vi "exv valves.vi"(0 "Large Gas Cluster":T8, 1 "Medium Gas Cluster":T7, 3 "Small Gas Cluster":T6, 4 "Large Liquid Cluster":T5, 5 "Medium Liquid Cluster":T4, 7 "Small Liquid Cluster":T3, 8 "Tonnage":dbl, 9 "Desired Psuc":dbl, 10 "Reinitialize Controller P":bool, 11 "Controller Toggle P":bool, 12 "Tonnage Threshold":dbl=40.0 format="%#_13g", 13 "Desired Tsuc":dbl, 14 "Delta P Threshold":dbl=5.0 format="%#_13g", 15 "Current Psuc":dbl format="%#_13g", 16 "Delta T Threshold":dbl=5.0 format="%#_13g", 17 "Current Tsuc":dbl format="%#_13g", 18 "Reinitialize Controller T":bool, 19 "Controller Toggle T":bool) -> (20 "Gas Valves Output":T2, 27 "Liquid Valves Output":T1)   [LabVIEW 2017]
doc: "Control logic for all controllers on liquid and gas lines. Thresholding procedure that determines which controller should be operating based on current process variable. Passes the chosen controller to the PID vi's"
panel:
  out "output to valve 3":dbl
  out "output to valve 2":dbl
  out "output to valve":dbl
  out "PID gains out small Liquid":T9
  out "Small Liquid Tuning Complete":bool
  out "Small Liquid Output":dbl(slide) scale=0.0..100.0 scale format="%#_3g"
  out "PID gains out Medium Liquid":T9
  out "Medium Liquid Tuning Complete":bool
  out "Medium Liquid Output":dbl(slide) scale=0.0..100.0 scale format="%#_3g"
  out "PID gains out large liquid":T9
  out "Large Liquid Tuning Complete":bool
  out "Large Liquid Output":dbl(slide) scale=0.0..100.0 scale format="%#_3g"
  out "PID gains out small gas":T9
  out "Small Gas Tuning Complete":bool
  out "Small Gas Output":dbl(slide) scale=0.0..100.0 scale format="%#_3g"
  out "PID gains out Medium gas":T9
  out "Medium Gas Tuning Complete":bool
  out "Medium Gas Output":dbl(slide) scale=0.0..100.0 scale format="%#_3g"
  out "PID gains out large gas":T9
  out "Large Gas Tuning Complete":bool
  out "Large Gas Output":dbl(slide) scale=0.0..100.0 scale format="%#_3g"
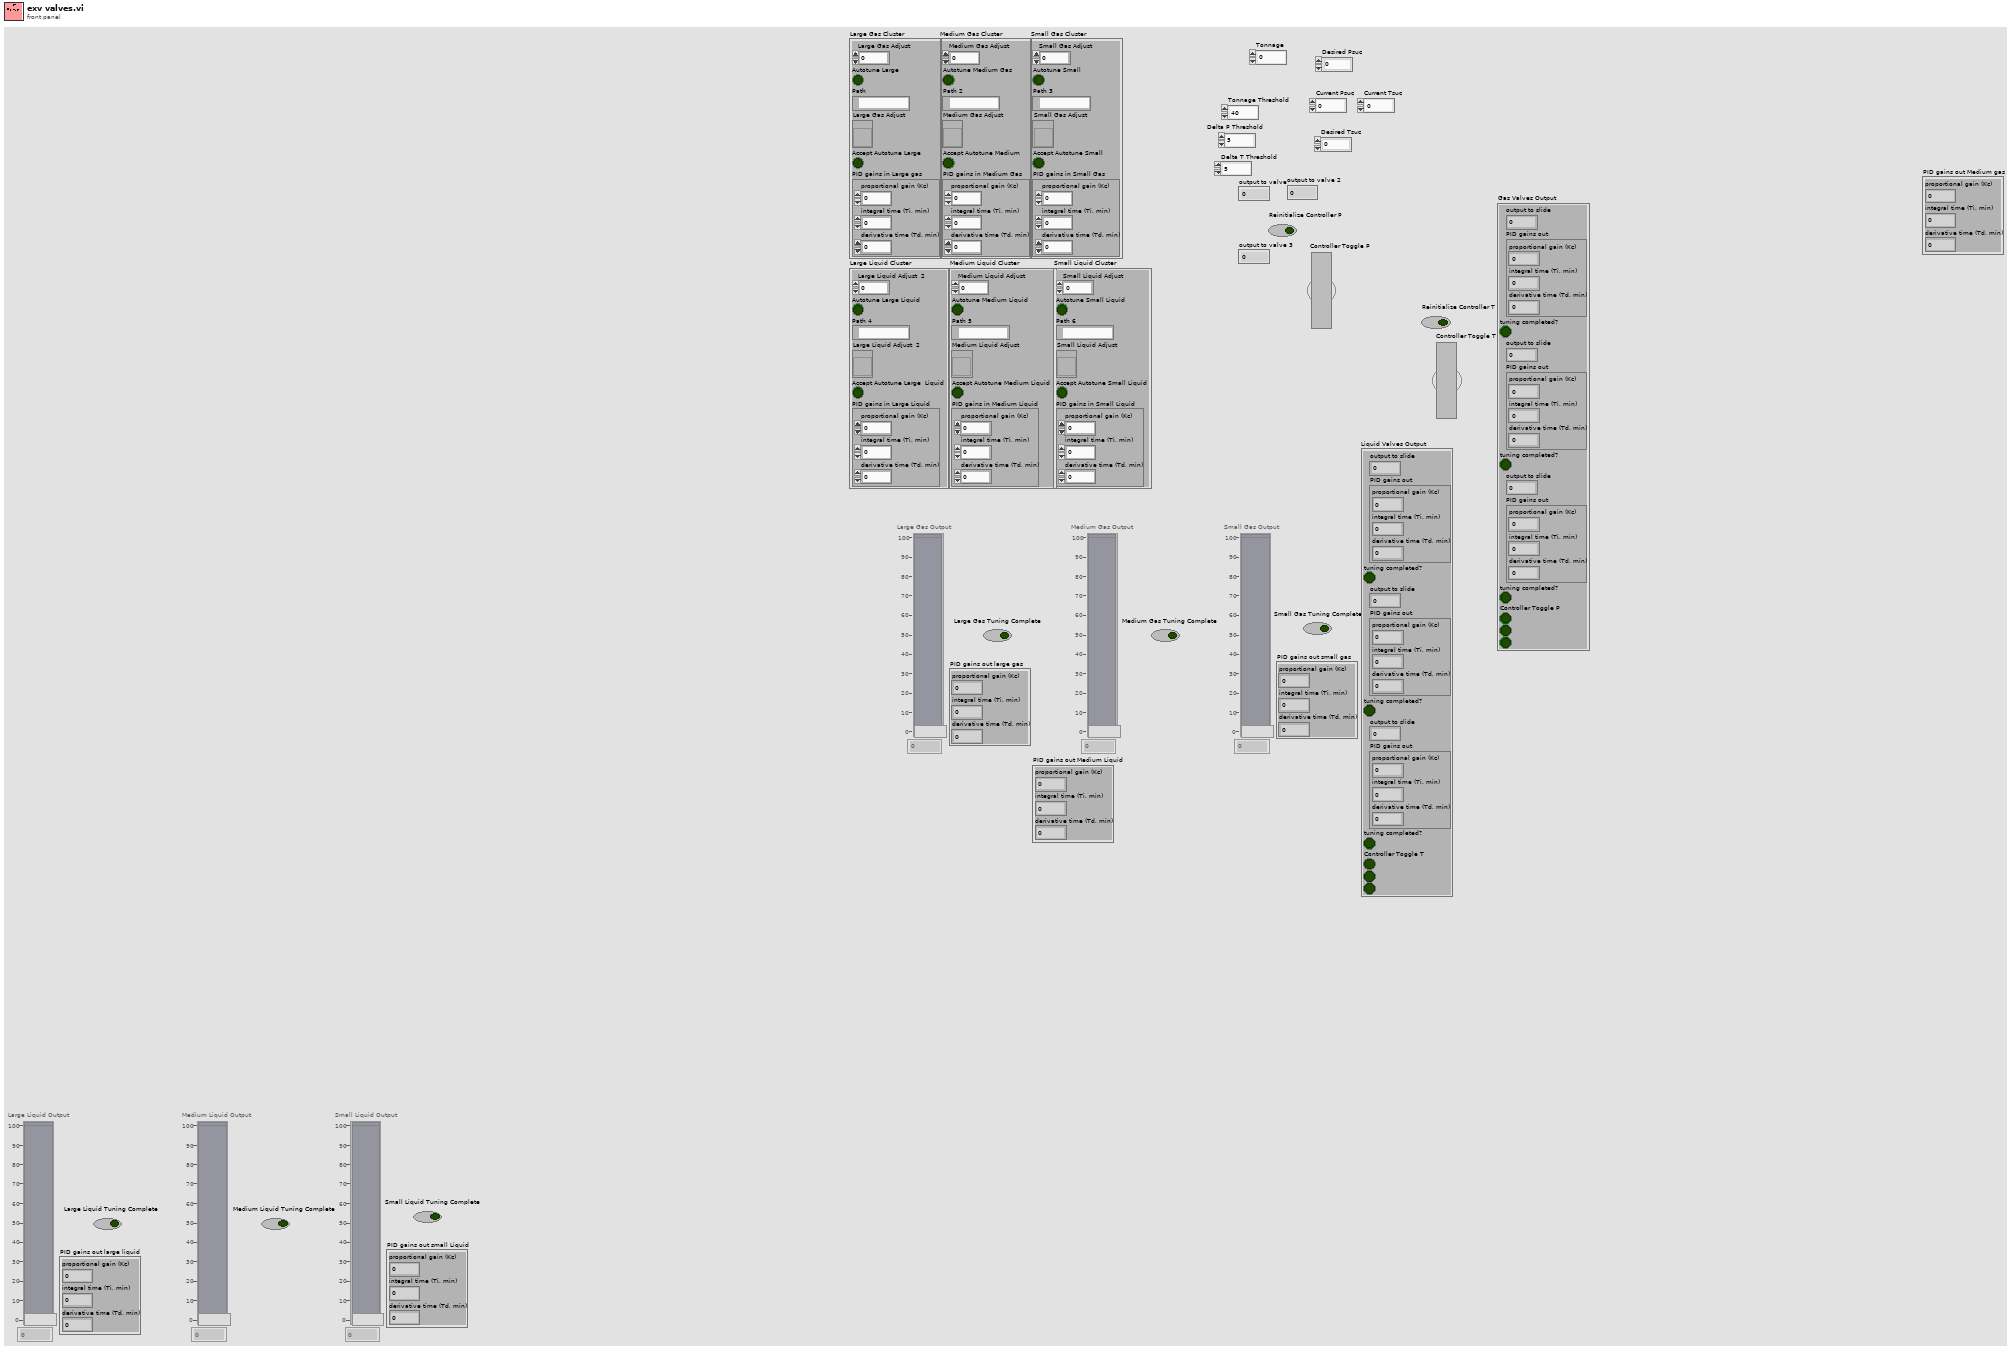
[diagram p1: front panel]
types:
  T1 = cluster{"output to slide":dbl, "PID gains out":cluster{"proportional gain (Kc)":dbl, "integral time (Ti, min)":dbl, "derivative time (Td, min)":dbl}, "tuning completed?":bool, "output to slide":dbl, "PID gains out":cluster{"proportional gain (Kc)":dbl, "integral time (Ti, min)":dbl, "derivative time (Td, min)":dbl}, "tuning completed?":bool, "output to slide":dbl, "PID gains out":cluster{"proportional gain (Kc)":dbl, "integral time (Ti, min)":dbl, "derivative time (Td, min)":dbl}, "tuning completed?":bool, "Controller Toggle T":bool, bool, bool}
  T2 = cluster{"output to slide":dbl, "PID gains out":cluster{"proportional gain (Kc)":dbl, "integral time (Ti, min)":dbl, "derivative time (Td, min)":dbl}, "tuning completed?":bool, "output to slide":dbl, "PID gains out":cluster{"proportional gain (Kc)":dbl, "integral time (Ti, min)":dbl, "derivative time (Td, min)":dbl}, "tuning completed?":bool, "output to slide":dbl, "PID gains out":cluster{"proportional gain (Kc)":dbl, "integral time (Ti, min)":dbl, "derivative time (Td, min)":dbl}, "tuning completed?":bool, "Controller Toggle P":bool, bool, bool}
  T3 = cluster{"Small Liquid Adjust ":dbl, "Autotune Small Liquid":bool, "Path 6":path, "Small Liquid Adjust ":refnum<vi>, "Accept Autotune Small Liquid":bool, "PID gains in Small Liquid":cluster{"proportional gain (Kc)":dbl, "integral time (Ti, min)":dbl, "derivative time (Td, min)":dbl}}
  T4 = cluster{"Medium Liquid Adjust":dbl, "Autotune Medium Liquid":bool, "Path 5":path, "Medium Liquid Adjust":refnum<vi>, "Accept Autotune Medium Liquid":bool, "PID gains in Medium Liquid":cluster{"proportional gain (Kc)":dbl, "integral time (Ti, min)":dbl, "derivative time (Td, min)":dbl}}
  T5 = cluster{"Large Liquid Adjust  2":dbl, "Autotune Large Liquid":bool, "Path 4":path, "Large Liquid Adjust  2":refnum<vi>, "Accept Autotune Large  Liquid":bool, "PID gains in Large Liquid":cluster{"proportional gain (Kc)":dbl, "integral time (Ti, min)":dbl, "derivative time (Td, min)":dbl}}
  T6 = cluster{"Small Gas Adjust":dbl, "Autotune Small":bool, "Path 3":path, "Small Gas Adjust":refnum<vi>, "Accept Autotune Small":bool, "PID gains in Small Gas ":cluster{"proportional gain (Kc)":dbl, "integral time (Ti, min)":dbl, "derivative time (Td, min)":dbl}}
  T7 = cluster{"Medium Gas Adjust":dbl, "Autotune Medium Gas":bool, "Path 2":path, "Medium Gas Adjust":refnum<vi>, "Accept Autotune Medium":bool, "PID gains in Medium Gas":cluster{"proportional gain (Kc)":dbl, "integral time (Ti, min)":dbl, "derivative time (Td, min)":dbl}}
  T8 = cluster{"Large Gas Adjust ":dbl, "Autotune Large":bool, "Path":path, "Large Gas Adjust ":refnum<vi>, "Accept Autotune Large ":bool, "PID gains in Large gas":cluster{"proportional gain (Kc)":dbl, "integral time (Ti, min)":dbl, "derivative time (Td, min)":dbl}}
  T9 = cluster{"proportional gain (Kc)":dbl, "integral time (Ti, min)":dbl, "derivative time (Td, min)":dbl}
  T10 = enum8{"Enabled", "Disabled", "Disabled and Grayed Out"}
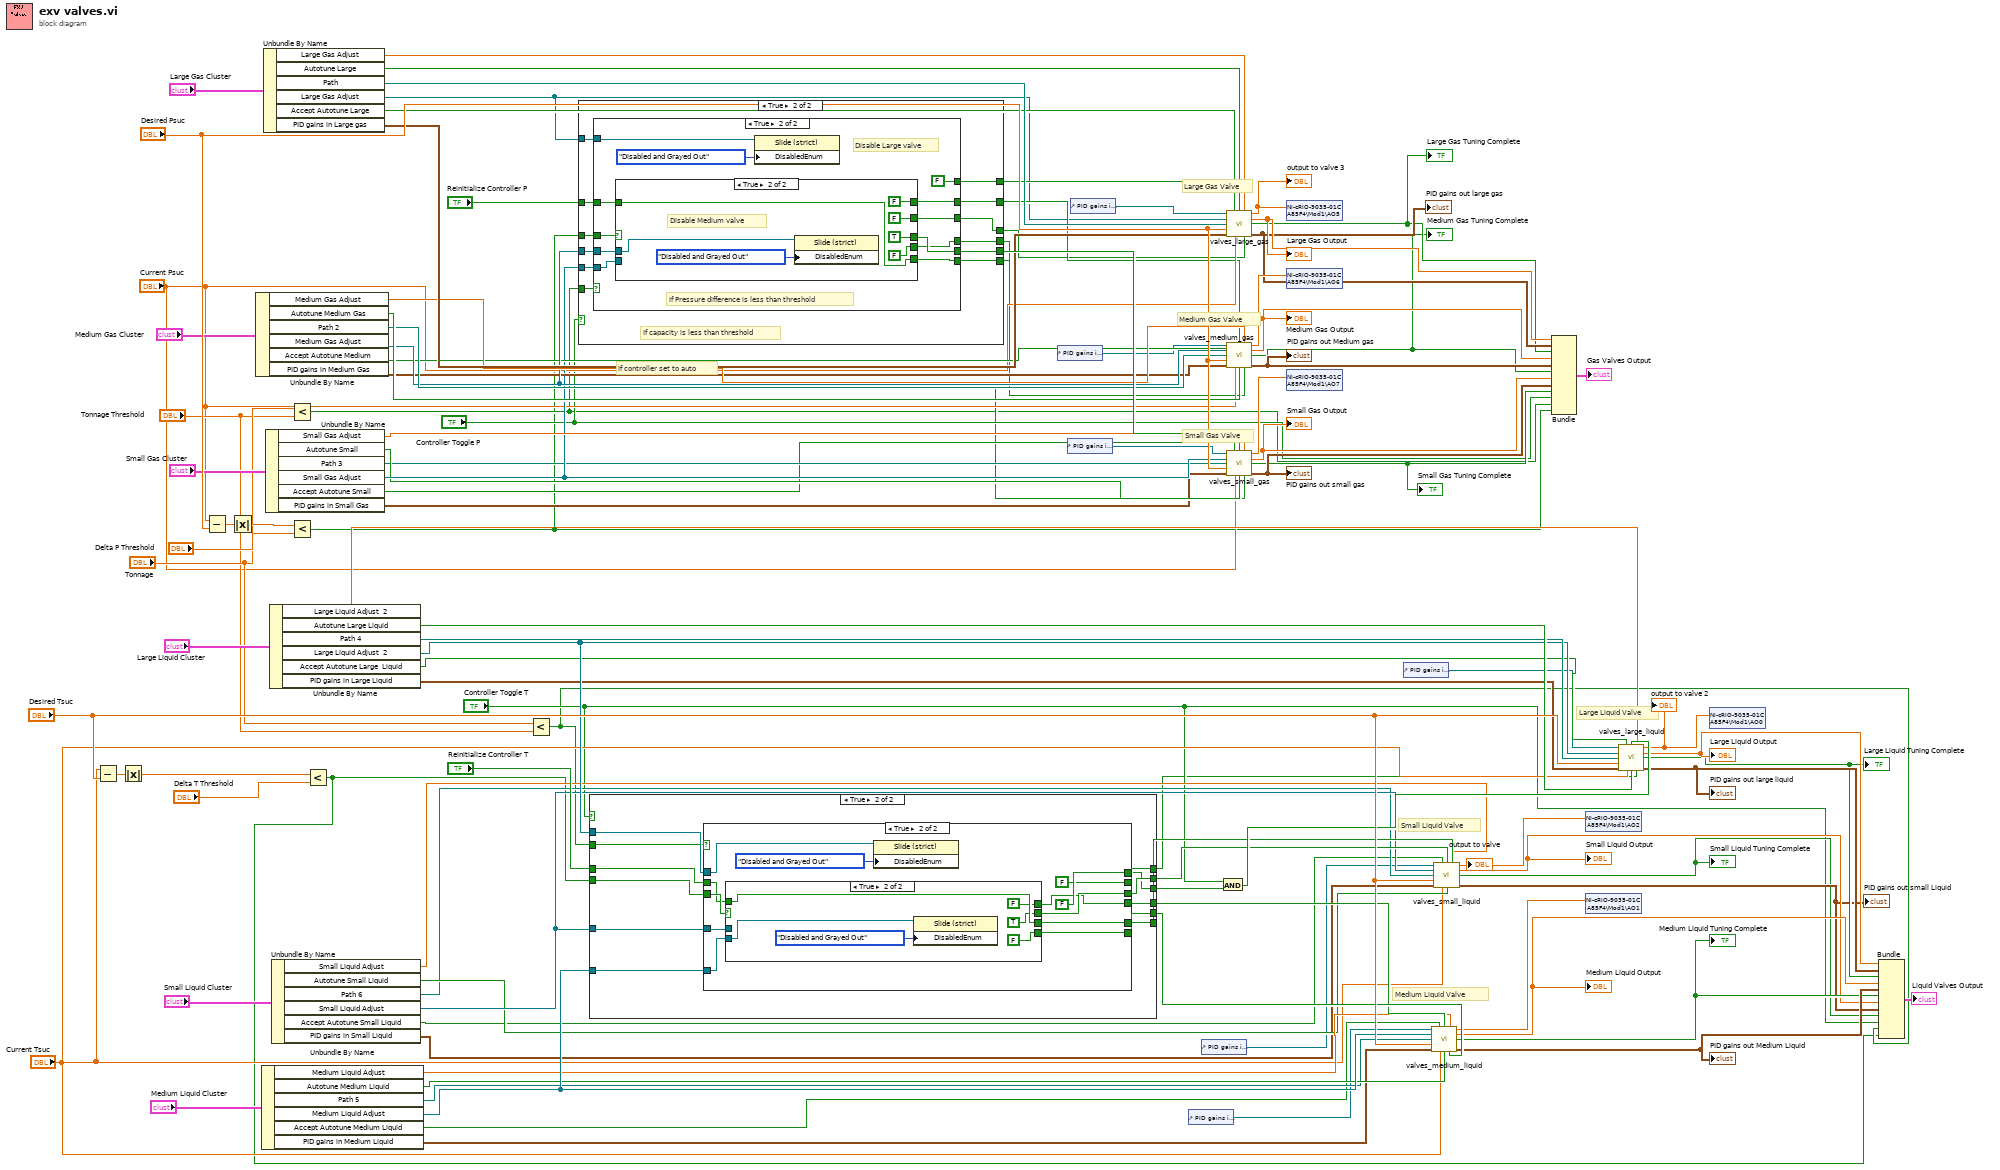
[diagram p0: block diagram]
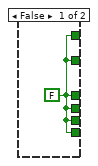
[diagram p2: hidden frame]
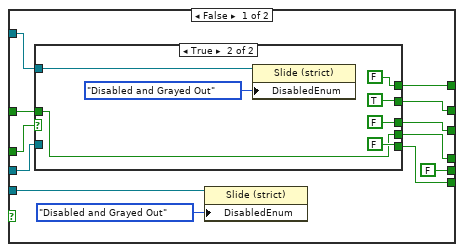
[diagram p3: hidden frame]
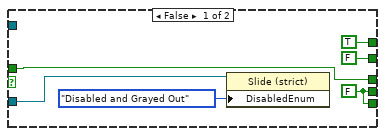
[diagram p4: hidden frame]
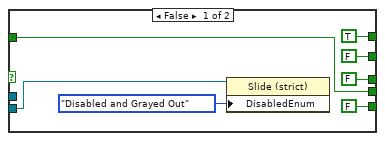
[diagram p5: hidden frame]
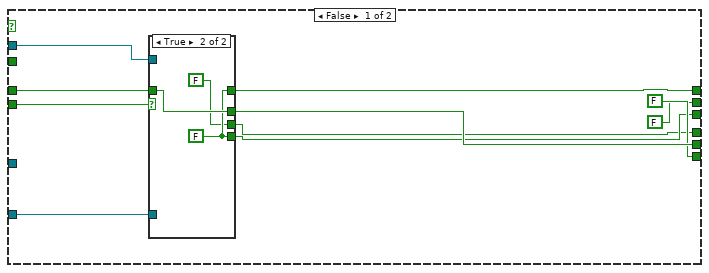
[diagram p6: hidden frame]
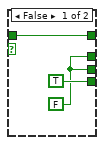
[diagram p7: hidden frame]
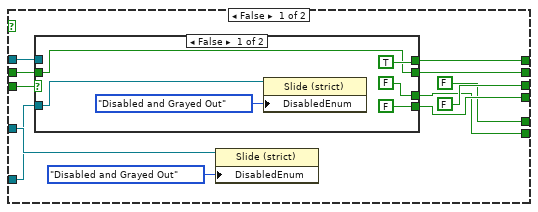
[diagram p8: hidden frame]
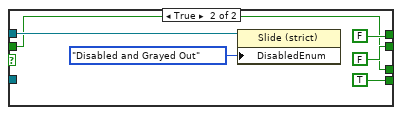
[diagram p9: hidden frame]
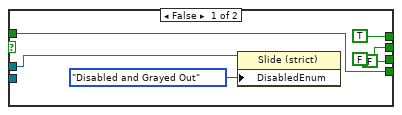
[diagram p10: hidden frame]
diagram:
  # "If controller set to auto"
  # "Large Liquid Valve"
  # "Medium Liquid Valve"
  # "Small Liquid Valve"
  # "Large Gas Valve"
  # "Medium Gas Valve"
  # "Small Gas Valve"
  n1 = Subtract(x="Current Tsuc", y="Desired Tsuc") -> (x-y=w86:dbl)
  n2 = Absolute Value(x=w86) -> (abs(x)=w85:dbl)
  n3 = Subtract(x="Current Psuc", y="Desired Psuc") -> (x-y=w101:dbl)
  n4 = Absolute Value(x=w101) -> (abs(x)=w100:dbl)
  n5 = Unbundle By Name("Medium Gas Cluster") -> ("Medium Gas Adjust"=w63:dbl, "Autotune Medium Gas"=w62:bool, "Path 2"=w61:path, "Medium Gas Adjust"=w60:refnum<vi>, "Accept Autotune Medium"=w59:bool, "PID gains in Medium Gas"=w58:T9)
  n6 = Unbundle By Name("Medium Liquid Cluster") -> ("Medium Liquid Adjust"=w38:dbl, "Autotune Medium Liquid"=w37:bool, "Path 5"=w36:path, "Medium Liquid Adjust"=w39:refnum<vi>, "Accept Autotune Medium Liquid"=w35:bool, "PID gains in Medium Liquid"=w34:T9)
  n7 = Unbundle By Name("Large Gas Cluster") -> ("Large Gas Adjust"=w10:dbl, "Autotune Large"=w69:bool, "Path"=w68:path, "Large Gas Adjust"=w7:refnum<vi>, "Accept Autotune Large"=w67:bool, "PID gains in Large gas"=w66:T9)
  n8 = Unbundle By Name("Small Gas Cluster") -> ("Small Gas Adjust"=w55:dbl, "Autotune Small"=w53:bool, "Path 3"=w52:path, "Small Gas Adjust"=w54:refnum<vi>, "Accept Autotune Small"=w51:bool, "PID gains in Small Gas"=w50:T9)
  n9 = Unbundle By Name("Large Liquid Cluster") -> ("Large Liquid Adjust  2"=w47:dbl, "Autotune Large Liquid"=w46:bool, "Path 4"=w45:path, "Large Liquid Adjust  2"=w44:refnum<vi>, "Accept Autotune Large  Liquid"=w43:bool, "PID gains in Large Liquid"=w42:T9)
  n10 = Unbundle By Name("Small Liquid Cluster") -> ("Small Liquid Adjust"=w30:dbl, "Autotune Small Liquid"=w29:bool, "Path 6"=w28:path, "Small Liquid Adjust"=w31:refnum<vi>, "Accept Autotune Small Liquid"=w27:bool, "PID gains in Small Liquid"=w26:T9)
  n11 = Less?(x="Tonnage", y="Tonnage Threshold") -> (x < y?=w4:bool)
  n12 = Less?(x=w100, y="Delta P Threshold") -> (x < y?=w3:bool)
  n13 = Less?(x=w85, y="Delta T Threshold") -> (x < y?=w1:bool)
  n14 = Less?(x="Tonnage", y="Tonnage Threshold") -> (x < y?=w2:bool)
  n15 = case shown="True" "Controller Toggle P" {
    tunnel: "Reinitialize Controller P" -> [_ w120]
    tunnel: w3 -> [_ w119]
    tunnel: [w108 w118] -> w6
    tunnel: [w108 w117] -> w99
    tunnel: w7 -> [_ w116]
    tunnel: w60 -> [_ w115]
    tunnel: w54 -> [_ w114]
    tunnel: [w108 w113] -> w15
    tunnel: [w108 w112] -> w14
    tunnel: w4 -> [_ w111]
    tunnel: [w108 w110] -> w9
    tunnel: [w108 w109] -> w8
    frame False {
      w108 = FALSE ("Reinitialize Controller P")
    }
    frame True {
      # "If capacity is less than threshold"
      n16 = case shown="True" w111 {
        tunnel: w116 -> [w122 w150]
        tunnel: w120 -> [w129 w153]
        tunnel: w114 -> [w132 w152]
        tunnel: [w126 FALSE ("Reinitialize Controller P")] -> w112
        tunnel: w119 -> [w130 w155]
        tunnel: w115 -> [w128 w154]
        tunnel: [w123 w146] -> w118
        tunnel: [w121 w147] -> w113
        tunnel: [FALSE ("Reinitialize Controller P") w151] -> w117
        tunnel: [w125 w149] -> w110
        tunnel: [w124 w148] -> w109
        frame False {
          n17 = case shown="True" w130 {
            tunnel: w129 -> [w134 w140]
            tunnel: w122 -> [_ w144]
            tunnel: w128 -> [w137 _]
            tunnel: [TRUE ("Reinitialize Controller P") FALSE ("Reinitialize Controller P")] -> w126
            tunnel: [FALSE ("Reinitialize Controller P") TRUE] -> w121
            tunnel: [w133 FALSE ("Reinitialize Controller P")] -> w125
            tunnel: [w134 FALSE ("Reinitialize Controller P")] -> w124
            tunnel: [w133 w140] -> w123
            frame False {
              w133 = FALSE ("Reinitialize Controller P")
              n18 = property on="Property Node" class="Slide (strict)"(reference=w137, "DisabledEnum"=T10."Disabled and Grayed Out" ("Disabled")) -> ()  [unwired: 1 in, 2 out]
            }
            frame True {
              n19 = property on="Property Node" class="Slide (strict)"(reference=w144, "DisabledEnum"=T10."Disabled and Grayed Out" ("Disabled")) -> ()  [unwired: 1 in, 2 out]
            }
          }
          n20 = property on="Property Node" class="Slide (strict)"(reference=w132, "DisabledEnum"=T10."Disabled and Grayed Out" ("Disabled")) -> ()  [unwired: 1 in, 2 out]
        }
        frame True {
          # "If Pressure difference is less than threshold"
          # "Disable Large valve"
          n21 = case shown="True" w155 {
            tunnel: w154 -> [_ w171]
            tunnel: w153 -> [w159 w166]
            tunnel: [w159 FALSE ("Reinitialize Controller P")] -> w146
            tunnel: w152 -> [w161 _]
            tunnel: [TRUE ("Reinitialize Controller P") FALSE ("Reinitialize Controller P")] -> w147
            tunnel: [FALSE ("Reinitialize Controller P") TRUE ("Reinitialize Controller P")] -> w151
            tunnel: [FALSE ("Reinitialize Controller P") w166] -> w149
            tunnel: [FALSE ("Reinitialize Controller P") FALSE ("Reinitialize Controller P")] -> w148
            frame False {
              n22 = property on="Property Node" class="Slide (strict)"(reference=w161, "DisabledEnum"=T10."Disabled and Grayed Out" ("Disabled")) -> ()  [unwired: 1 in, 2 out]
            }
            frame True {
              # "Disable Medium valve"
              n23 = property on="Property Node" class="Slide (strict)"(reference=w171, "DisabledEnum"=T10."Disabled and Grayed Out" ("Disabled")) -> ()  [unwired: 1 in, 2 out]
            }
          }
          n24 = property on="Property Node" class="Slide (strict)"(reference=w150, "DisabledEnum"=T10."Disabled and Grayed Out" ("Disabled")) -> ()  [unwired: 1 in, 2 out]
        }
      }
    }
  }
  n25 = case shown="True" "Controller Toggle T" {
    tunnel: w44 -> [w177 w199]
    tunnel: "Reinitialize Controller T" -> [w180 w196]
    tunnel: w31 -> [_ w189]
    tunnel: [w173 w190] -> w5
    tunnel: w1 -> [w181 w198]
    tunnel: w39 -> [w176 w197]
    tunnel: [FALSE ("Reinitialize Controller P") w195] -> w83
    tunnel: [w179 w193] -> w82
    tunnel: [w178 w191] -> w12
    tunnel: [w172 w188] -> w81
    tunnel: [FALSE ("Reinitialize Controller P") w194] -> w80
    tunnel: w2 -> [_ w192]
    frame False {
      n26 = case shown="True" w181 {
        tunnel: w180 -> [w184 w187]
        tunnel: [w182 w187] -> w179
        tunnel: [w184 w186] -> w178
        tunnel: w177 -> [_ _]
        tunnel: w176 -> [_ _]
        tunnel: [TRUE ("Reinitialize Controller P") w186] -> w173
        tunnel: [w182 FALSE] -> w172
        frame False {
          w182 = FALSE ("Reinitialize Controller P")
        }
        frame True {
          w186 = FALSE ("Reinitialize Controller P")
        }
      }
    }
    frame True {
      n27 = case shown="True" w192 {
        tunnel: w199 -> [w207 w234]
        tunnel: w198 -> [w201 w233]
        tunnel: w197 -> [w208 w232]
        tunnel: w196 -> [w205 w231]
        tunnel: [FALSE ("Reinitialize Controller T") w230] -> w195
        tunnel: w189 -> [w210 w229]
        tunnel: [FALSE ("Reinitialize Controller P") w228] -> w194
        tunnel: [w200 w227] -> w193
        tunnel: [w204 FALSE ("Reinitialize Controller P")] -> w191
        tunnel: [w206 FALSE ("Reinitialize Controller P")] -> w190
        tunnel: [w203 w224] -> w188
        frame False {
          n28 = case shown="False" w201 {
            tunnel: w208 -> [w216 _]
            tunnel: w207 -> [_ w222]
            tunnel: [w213 FALSE ("Reinitialize Controller P")] -> w204
            tunnel: [TRUE ("Reinitialize Controller P") FALSE ("Reinitialize Controller P")] -> w206
            tunnel: [FALSE ("Reinitialize Controller P") TRUE ("Reinitialize Controller P")] -> w203
            tunnel: [FALSE ("Reinitialize Controller P") w218] -> w200
            tunnel: w205 -> [w213 w218]
            frame False {
              n29 = property on="Property Node" class="Slide (strict)"(reference=w216, "DisabledEnum"=T10."Disabled and Grayed Out" ("Disabled")) -> ()  [unwired: 1 in, 2 out]
            }
            frame True {
              n30 = property on="Property Node" class="Slide (strict)"(reference=w222, "DisabledEnum"=T10."Disabled and Grayed Out" ("Disabled")) -> ()  [unwired: 1 in, 2 out]
            }
          }
          n31 = property on="Property Node" class="Slide (strict)"(reference=w210, "DisabledEnum"=T10."Disabled and Grayed Out" ("Disabled")) -> ()  [unwired: 1 in, 2 out]
        }
        frame True {
          n32 = case shown="True" w233 {
            tunnel: w232 -> [_ w246]
            tunnel: w231 -> [w241 w245]
            tunnel: [FALSE ("Reinitialize Controller T") w245] -> w230
            tunnel: [w241 FALSE ("Reinitialize Controller P")] -> w227
            tunnel: w229 -> [w239 _]
            tunnel: [FALSE ("Reinitialize Controller P") TRUE ("Reinitialize Controller P")] -> w228
            tunnel: [TRUE ("Reinitialize Controller P") FALSE ("Reinitialize Controller P")] -> w224
            frame False {
              n33 = property on="Property Node" class="Slide (strict)"(reference=w239, "DisabledEnum"=T10."Disabled and Grayed Out" ("Disabled")) -> ()  [unwired: 1 in, 2 out]
            }
            frame True {
              n34 = property on="Property Node" class="Slide (strict)"(reference=w246, "DisabledEnum"=T10."Disabled and Grayed Out" ("Disabled")) -> ()  [unwired: 1 in, 2 out]
            }
          }
          n35 = property on="Property Node" class="Slide (strict)"(reference=w234, "DisabledEnum"=T10."Disabled and Grayed Out" ("Disabled")) -> ()  [unwired: 1 in, 2 out]
        }
      }
    }
  }
  n36 = control-ref of="PID gains in Medium Gas"() -> (w57:refnum<vi>)
  n37 = control-ref of="PID gains in Small Gas"() -> (w49:refnum<vi>)
  n38 = control-ref of="PID gains in Large gas"() -> (w65:refnum<vi>)
  n39 = control-ref of="PID gains in Medium Liquid"() -> (w33:refnum<vi>)
  n40 = control-ref of="PID gains in Small Liquid"() -> (w25:refnum<vi>)
  n41 = And(x="Controller Toggle T", y=w5) -> (x .and. y?=w84:bool)
  n42 = call "valves_large_gas.vi"("PID Gains Cluster Ref"=w65, "Accept Autotune"=w67, "Controller Toggle (Manual Mode)"=w14, "Valve Manual Adjust"=w10, "Slide Refnum in"=w7, "file (use dialog)"=w68, "Desired Setpoint"="Desired Psuc", "PID gains"=w66, "Current Process Variable Value"="Current Psuc", "autotune? (F)"=w69, "Reinitialize Controller"=w8) -> ("output to valve"=w107:dbl, "output to slide"=w98:dbl, "tuning completed?"=w96:bool, "PID gains out"=w97:T9)  [unwired: 1 out]
  "Large Gas Output" <- w98
  "Large Gas Tuning Complete" <- w96
  "PID gains out large gas" <- w97
  "output to valve 3" <- w107
  n43 = call "valves_medium_gas.vi"("PID Gains Cluster Ref"=w57, "Accept Autotune"=w59, "Controller Toggle (Manual Mode)"=w15, "Valve Manual Adjust"=w63, "Slide Refnum in"=w60, "file (use dialog)"=w61, "Desired Setpoint"="Desired Psuc", "PID gains"=w58, "Current Process Variable Value"="Current Psuc", "autotune? (F)"=w62, "Reinitialize Controller"=w6) -> ("output to valve"=w106:dbl, "output to slide"=w95:dbl, "tuning completed?"=w93:bool, "PID gains out"=w94:T9)  [unwired: 1 out]
  "Medium Gas Output" <- w95
  "Medium Gas Tuning Complete" <- w93
  "PID gains out Medium gas" <- w94
  n44 = call "valves_small_gas.vi"("PID Gains Cluster Ref"=w49, "Accept Autotune"=w51, "Controller Toggle (Manual Mode)"=w99, "Valve Manual Adjust"=w55, "Slide Refnum in"=w54, "file (use dialog)"=w52, "Desired Setpoint"="Desired Psuc", "PID gains"=w50, "Current Process Variable Value"="Current Psuc", "autotune? (F)"=w53, "Reinitialize Controller"=w9) -> ("output to valve"=w105:dbl, "output to slide"=w92:dbl, "tuning completed?"=w90:bool, "PID gains out"=w91:T9)  [unwired: 1 out]
  "Small Gas Output" <- w92
  "Small Gas Tuning Complete" <- w90
  "PID gains out small gas" <- w91
  n45 = shared-variable "NI-cRIO-9035-01CA85F4\\Mod1\\AO5"(w107) -> ()  [unwired: 1 in, 1 out]
  n46 = shared-variable "NI-cRIO-9035-01CA85F4\\Mod1\\AO6"(w106) -> ()  [unwired: 1 in, 1 out]
  n47 = shared-variable "NI-cRIO-9035-01CA85F4\\Mod1\\AO7"(w105) -> ()  [unwired: 1 in, 1 out]
  n48 = control-ref of="PID gains in Large Liquid"() -> (w41:refnum<vi>)
  n49 = call "valves_medium_liquid.vi"("PID Gains Cluster Ref"=w33, "Accept Autotune"=w35, "Controller Toggle (Manual Mode)"=w81, "Valve Manual Adjust"=w38, "Slide Refnum in"=w39, "file (use dialog)"=w36, "Desired Setpoint"="Desired Tsuc", "PID gains"=w34, "Current Process Variable Value"="Current Tsuc", "autotune? (F)"=w37, "Reinitialize Controller"=w82) -> ("output to valve"=w18:dbl, "output to slide"=w76:dbl, "tuning completed?"=w74:bool, "PID gains out"=w75:T9)  [unwired: 1 out]
  "Medium Liquid Output" <- w76
  "Medium Liquid Tuning Complete" <- w74
  "PID gains out Medium Liquid" <- w75
  n50 = call "valves_small_liquid.vi"("PID Gains Cluster Ref"=w25, "Accept Autotune"=w27, "Controller Toggle (Manual Mode)"=w80, "Valve Manual Adjust"=w30, "Slide Refnum in"=w31, "file (use dialog)"=w28, "Desired Setpoint"="Desired Tsuc", "PID gains"=w26, "Current Process Variable Value"="Current Tsuc", "autotune? (F)"=w29, "Reinitialize Controller"=w83) -> ("output to valve"=w16:dbl, "output to slide"=w73:dbl, "tuning completed?"=w71:bool, "PID gains out"=w72:T9)  [unwired: 1 out]
  "Small Liquid Output" <- w73
  "Small Liquid Tuning Complete" <- w71
  "PID gains out small Liquid" <- w72
  "output to valve" <- w16
  n51 = Bundle("output to slide"=w98, "PID gains out"=w97, "tuning completed?"=w96, "output to slide"=w95, "PID gains out"=w94, "tuning completed?"=w93, "output to slide"=w92, "PID gains out"=w91, "tuning completed?"=w90, "Controller Toggle P"="Controller Toggle P", w4, w3) -> (→"Gas Valves Output":T2)  [unwired: 1 in]
  n52 = shared-variable "NI-cRIO-9035-01CA85F4\\Mod1\\AO2"(w16) -> ()  [unwired: 1 in, 1 out]
  n53 = shared-variable "NI-cRIO-9035-01CA85F4\\Mod1\\AO1"(w18) -> ()  [unwired: 1 in, 1 out]
  n54 = call "valves_large_liquid.vi"("PID Gains Cluster Ref"=w41, "Accept Autotune"=w43, "Controller Toggle (Manual Mode)"=w84, "Valve Manual Adjust"=w47, "Slide Refnum in"=w44, "file (use dialog)"=w45, "Desired Setpoint"="Desired Tsuc", "PID gains"=w42, "Current Process Variable Value"="Current Tsuc", "autotune? (F)"=w46, "Reinitialize Controller"=w12) -> ("output to valve"=w17:dbl, "output to slide"=w79:dbl, "tuning completed?"=w77:bool, "PID gains out"=w78:T9)  [unwired: 1 out]
  "Large Liquid Output" <- w79
  "Large Liquid Tuning Complete" <- w77
  "PID gains out large liquid" <- w78
  "output to valve 2" <- w17
  n55 = shared-variable "NI-cRIO-9035-01CA85F4\\Mod1\\AO0"(w17) -> ()  [unwired: 1 in, 1 out]
  n56 = Bundle("output to slide"=w79, "PID gains out"=w78, "tuning completed?"=w77, "output to slide"=w76, "PID gains out"=w75, "tuning completed?"=w74, "output to slide"=w73, "PID gains out"=w72, "tuning completed?"=w71, "Controller Toggle T"="Controller Toggle T", w2, w1) -> (→"Liquid Valves Output":T1)  [unwired: 1 in]
